vi "Returning Values By Reference Array Of Complex Struct.vi"(8 "error in (no error)":errorcluster, 10 "length":i32, 11 "triangles":T1) -> (0 "error out":errorcluster, 2 "name":string, 3 "triangles out":T1)   [LabVIEW 2009, in "LabVIEWWrapper_PassingDataSampleDLL.lvlib"]
doc: "void ReturningValuesByReference_ArrayOfComplexStruct (struct complexStructPolygon **triangles, int length);"
uses:
  <vilib>/Utility/importsl/GetValueByPointer/GetValueByPointer.xnode
  <vilib>/Utility/importsl/GetValueByPointer/datatype.ctl
  LabVIEWWrapper_PassingDataSampleDLL.lvlib
  PassingDataSampleDLL.dll
  Program Files (x86)/National Instruments/LabVIEW 2009/resource/lvimptsl.dll
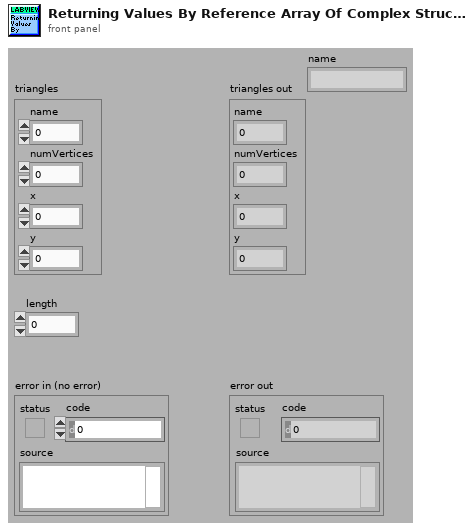
[diagram p1: front panel]
types:
  T1 = cluster{"name":u32, "numVertices":i32, "x":i32, "y":i32}
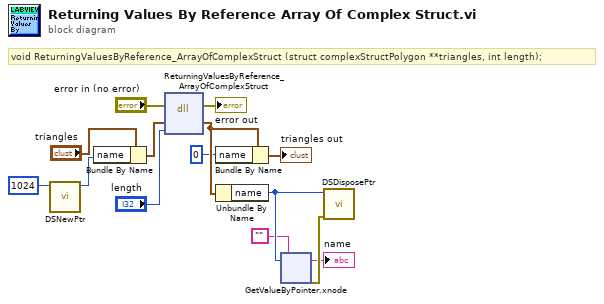
[diagram p0: block diagram]
diagram:
  # "void ReturningValuesByReference_ArrayOfComplexStruct (struct complexStructPolygon **triangles, int length);"
  n1 = call <vilib>:"DSNewPtr.vi"("Size"=u64 1024) -> ("Pointer"=w12:u64)  [unwired: 9 in, 1 out]
  n2 = Bundle By Name(cluster="triangles", "name"=w12) -> (w11:T1)
  n3 = dll-call lib="C:/My Dropbox/Systems Engineering Application/SDK/C Integration/LabVIEWWrapper/PassingDataSampleDLL.*" fn="ReturningValuesByReference_ArrayOfComplexStruct"(error in="error in (no error)", "triangles"=w11, "length"="length") -> (error out=→"error out":errorcluster, "triangles"=w6:T1)  [unwired: 4 in, 1 out]
  n4 = Bundle By Name(cluster=w6, "name"=u32 0) -> (→"triangles out":T1)
  n5 = Unbundle By Name(w6) -> ("name"=w9:u32)
  n6 = xnode "GetValueByPointer.xnode"("Pointer"=w9, "InputType"="") -> ("Output"=→"name":string, "ErrorOut"=w10:errorcluster)  [unwired: 2 in]
  n7 = call <vilib>:"DSDisposePtr.vi"("error in (no error)"=w10, "Pointer"=w9) -> ()  [unwired: 9 in, 1 out]
